vi "LSX Set Speed Poti.vi"(8 "error in (no error)":errorcluster, 10 "bSpeedPoti":i32, 11 "lLSID":i32) -> (0 "error out":errorcluster, 3 "function return":i32)   [LabVIEW 2018, in "Tango.lvlib"]
doc: "TANGOAPI int TANGOCALL LSX_SetSpeedPoti (int lLSID, BOOL bSpeedPoti);"
uses:
  Tango.lvlib
  SubVIs/Tango_DLL.dll
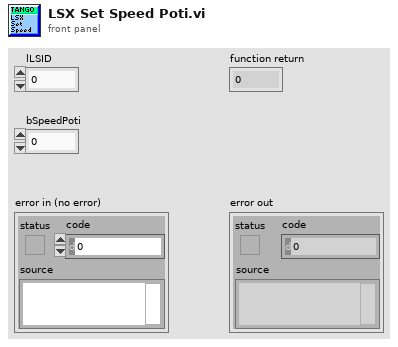
[diagram p1: front panel]
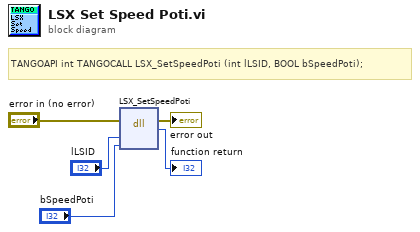
[diagram p0: block diagram]
diagram:
  # "TANGOAPI int TANGOCALL LSX_SetSpeedPoti (int lLSID, BOOL bSpeedPoti);"
  n1 = dll-call lib="C:/Users/Familie/Documents/LabviewIX81/lib/TANGO Stage/SubVIs/Tango_DLL.*" fn="LSX_SetSpeedPoti"(error in="error in (no error)", "lLSID"="lLSID", "bSpeedPoti"="bSpeedPoti") -> (error out=→"error out":errorcluster, →"function return":i32)  [unwired: 4 in, 1 out]
